vi "Init.vi"(8 "error in (no error)":errorcluster, 11 "Coca Actor in":refnum<class "Coca Actor.lvclass">) -> (0 "error out":errorcluster, 3 "Coca Actor out":refnum<class "Coca Actor.lvclass">)   [LabVIEW 2020, in "Coca Actor.lvlib" / "Coca Actor.lvclass"]
uses:
  Coca Actor.lvclass
  Coca Actor.lvclass/Coca Actor.ctl
  <vilib>/Utility/config.llb/Read Key (Double).vi
  <vilib>/Utility/config.llb/NI_LVConfig.lvlib
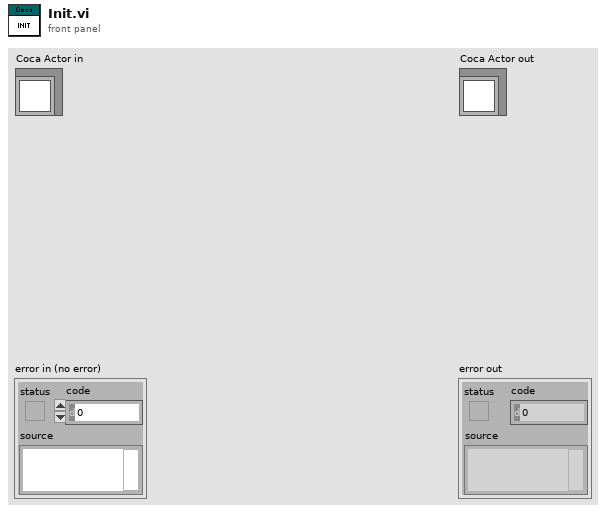
[diagram p1: front panel]
types:
  T1 = typedef "NI_LVConfig.lvlib/Config Data RefNum.ctl" = refnum<k1>
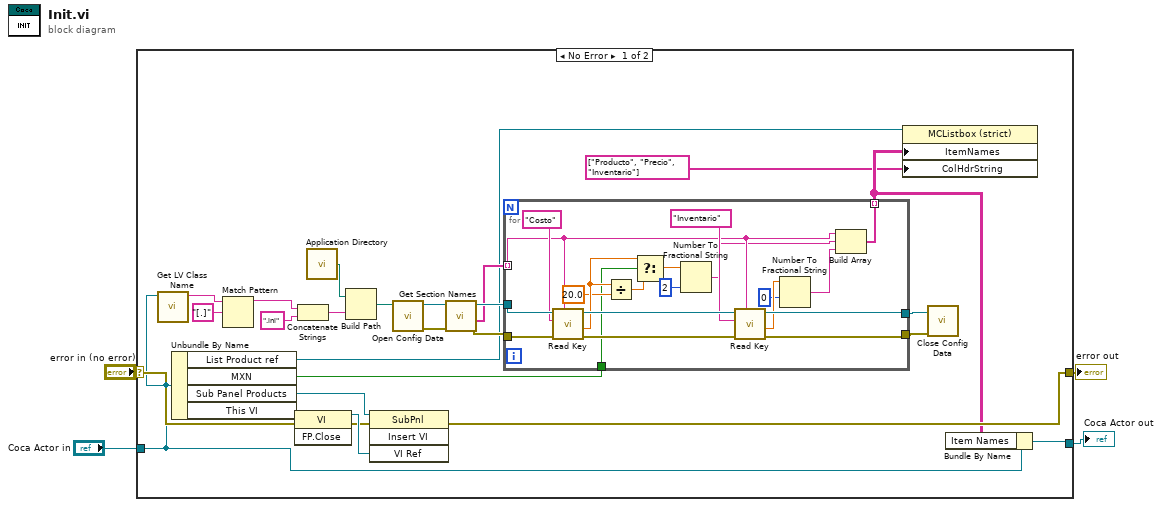
[diagram p0: block diagram]
diagram:
  n1 = case shown="No Error" "error in (no error)" {
    selector: "error in (no error)" -> [w11 w52]
    tunnel: [w10 w52] -> w3
    tunnel: [w5 w51] -> w1
    tunnel: "Coca Actor in" -> [w6 w51]
    frame No Error {
      n2 = call <vilib>:"Get LV Class Name.vi"("object"=w6) -> ("class name"=w20:string)  [unwired: 9 in, 1 out]
      n3 = Unbundle By Name(w6) -> ("List Product ref"=w9:refnum<vi>, "MXN"=w12:bool, "Sub Panel Products"=w30:refnum<vi>, "This VI"=w29:refnum<vi>)
      n4 = Match Pattern(string=w20, regular expression="[.]") -> (before substring=w19:string)  [unwired: 1 in, 3 out]
      n5 = invoke class="VI" method="FP.Close"(reference=w29, error in=w11) -> (reference out=w28:refnum<vi>, error out=w27:errorcluster)  [unwired: 1 in, 1 out]
      n6 = Concatenate Strings(w19, ".ini" ("string")) -> (w26:string)
      n7 = call <vilib>:"Application Directory.vi"() -> ("Application Directory"=w24:path)
      n8 = Build Path(base path=w24, name or relative path=w26) -> (appended path=w23:path)
      n9 = invoke class="SubPnl" method="Insert VI"(reference=w30, error in=w27, "VI Ref"=w28) -> (error out=w10:errorcluster)  [unwired: 1 in, 3 out]
      n10 = call <vilib>:"Open Config Data.vi"("configuration file path"=w23) -> ("error out"=w16:errorcluster, "refnum"=w17:T1)  [unwired: 8 in, 1 out]
      n11 = call <vilib>:"Get Section Names.vi"("error in (no error)"=w16, "refnum"=w17) -> ("error out"=w14:errorcluster, "section names"=w13:string[], "refnum out"=w15:T1)  [unwired: 7 in]
      n12 = for {
        tunnel: w15 -> [w50]
        tunnel: [w47] -> w22
        tunnel: [w46] -> w21
        tunnel: w14 -> [w43]
        tunnel: w13 -> [w42] mode=indexing
        tunnel: w12 -> [w35]
        tunnel: [w41] -> w8 mode=indexing
        n13 = call-poly <vilib>:"Read Key.vi"("section"=w42, "error in (no error)"=w43, "key"="Costo", "refnum"=w50) -> ("error out"=w49:errorcluster, "value"=w37:dbl, "refnum out"=w48:T1)  [unwired: 4 in, 1 out]
        n14 = Divide(x=w37, y=20.0) -> (x/y=w39:dbl)
        n15 = Select(t=w37, s=w35, f=w39) -> (s? t:f=w38:dbl)
        n16 = Number To Fractional String(number=w38, precision (6)=i16 2) -> (F-format string=w31:string)  [unwired: 2 in]
        n17 = call-poly <vilib>:"Read Key.vi"("section"=w42, "error in (no error)"=w49, "key"="Inventario", "refnum"=w48) -> ("error out"=w46:errorcluster, "value"=w34:dbl, "refnum out"=w47:T1)  [unwired: 4 in, 1 out]
        n18 = Number To Fractional String(number=w34, precision (6)=i16 0) -> (F-format string=w32:string)  [unwired: 2 in]
        n19 = Build Array(w42, w31, w32) -> (w41:string[])
      }
      n20 = property class="MCListbox (strict)"(reference=w9, "ItemNames"=w8, "ColHdrString"=string[] ["Producto", "Precio", "Inventario"] ("Column Header Strings[]")) -> ()  [unwired: 1 in, 2 out]
      n21 = call <vilib>:"Close Config Data.vi"("error in (no error)"=w21, "refnum"=w22) -> ()  [unwired: 8 in, 2 out]
      n22 = Bundle By Name(cluster=w6, "Item Names"=w8) -> (w5:refnum<class "Coca Actor.lvclass">)
    }
    frame Error {
    }
  }
  "error out" <- w3
  "Coca Actor out" <- w1
